vi "GoTo.vi"(6 "Busy":refnum<vi>, 8 "error in (no error)":errorcluster, 10 "Param":string, 11 "Rele in":refnum<class "Rele.lvclass">) -> (0 "error out":errorcluster, 2 "Response":string, 3 "Rele out":refnum<class "Rele.lvclass">)   [LabVIEW 2018, in "Rele.lvclass"]
uses:
  Rele.lvclass
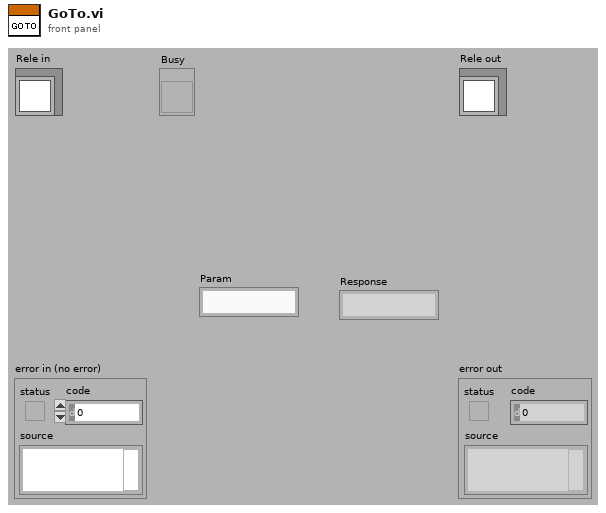
[diagram p1: front panel]
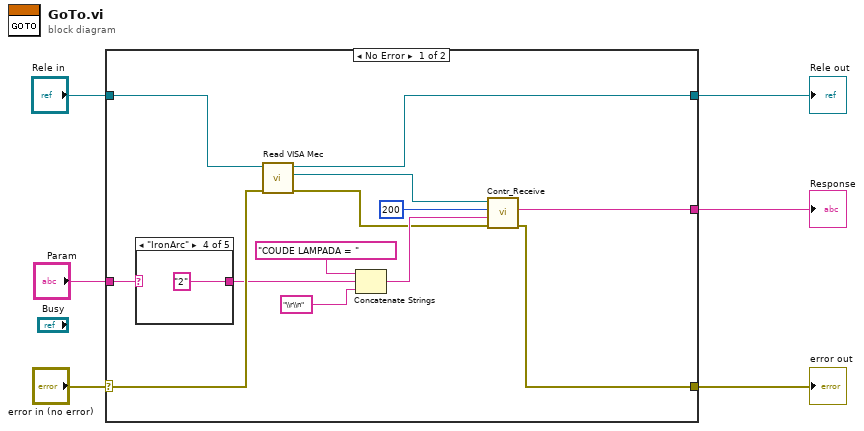
[diagram p0: block diagram]
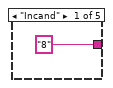
[diagram p2: hidden frame]
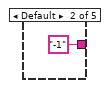
[diagram p3: hidden frame]
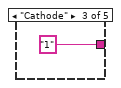
[diagram p4: hidden frame]
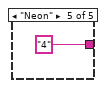
[diagram p5: hidden frame]
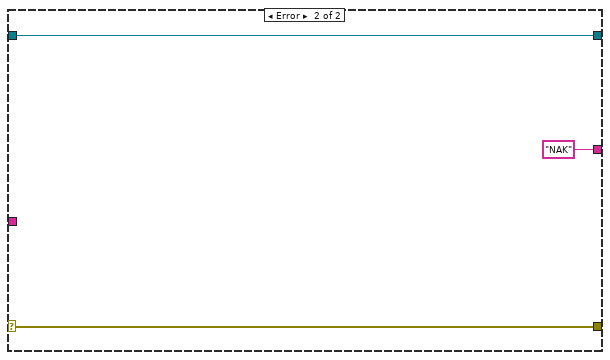
[diagram p6: hidden frame]
diagram:
  n1 = case shown="No Error" "error in (no error)" {
    selector: "error in (no error)" -> [w10 w26]
    tunnel: "Rele in" -> [w14 w27]
    tunnel: [w13 w27] -> w4
    tunnel: [w15 w26] -> w3
    tunnel: "Param" -> [w8 _]
    tunnel: [w9 "NAK" ("Response from SIFS")] -> w1
    frame No Error {
      n2 = case shown="\"IronArc\"" w8 {
        tunnel: ["8" "-1" "1" "2" "4"] -> w7
        frame "Incand" {
        }
        frame Default {
        }
        frame "Cathode" {
        }
        frame "IronArc" {
        }
        frame "Neon" {
        }
      }
      n3 = call-dynamic "Read VISA Mec.vi"("error in (no error)"=w10, "Controlador in"=w14) -> ("error out"=w11:errorcluster, "VISA Mec"=w12:refnum<visa-resource-name>, "Controlador out"=w13:refnum<class "Rele.lvclass">)  [unwired: 7 in]
      n4 = Concatenate Strings("COUDE LAMPADA = " ("Command to SIFS"), w7, "\\r\\n" ("string")) -> (w19:string)
      n5 = call "Contr_Receive.vi"("error in"=w11, "Command to SIFS"=w19, "wait after tx"=u32 200, "VISA resource name"=w12) -> ("error out"=w15:errorcluster, "Response from SIFS"=w9:string)  [unwired: 2 out]
    }
    frame Error {
    }
  }
  "error out" <- w3
  "Rele out" <- w4
  "Response" <- w1
